vi "ImageTest.vi"() -> ()   [LabVIEW 2017]
panel:
  out "Number of Particles (Particle Analysis 1)":i32
  out "Image Out 2":T1(plugin-control)
  in  "Stop (F)":bool
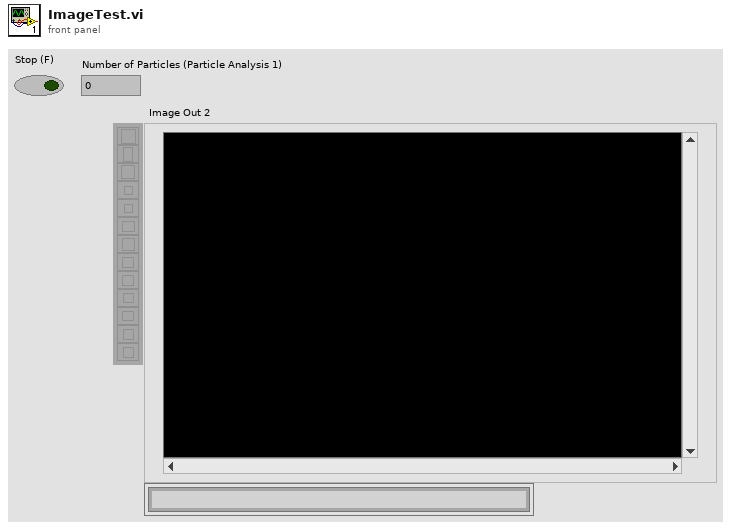
[diagram p1: front panel]
types:
  T1 = typedef "IMAQ Image.ctl" = refnum<image>
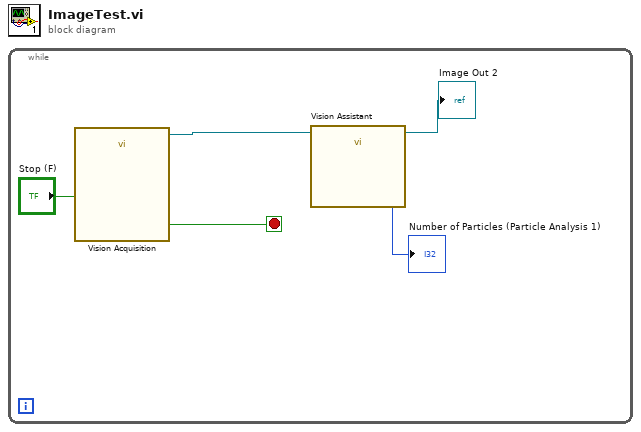
[diagram p0: block diagram]
diagram:
  n1 = while {
    stop <- w4 stop-if-true
    n2 = call "Vision Acquisition"("Stop (F)"="Stop (F)") -> ("Image Out"=w3:T1, "Stopped"=w4:bool)  [unwired: 24 in, 1 out]
    n3 = call "Vision Assistant"("Image In"=w3) -> ("Image Out"=→"Image Out 2":T1, "Number of Particles (Particle Analysis 1)"=→"Number of Particles (Particle Analysis 1)":i32)  [unwired: 24 in, 1 out]
  }
